vi "FindMutationByVerIndex.vi"(8 "error in (no error)":errorcluster, 9 "Old Name Index":u8, 10 "Library Version":T3, 11 "Mutation History":T4 {"LabVIEW Version" format="%.0x"}) -> (0 "error out":errorcluster, 1 "BlueSerializableVersion":T1, 2 "Mutation Record":T2 {"LabVIEW Version" format="%.0x"})   [LabVIEW 2019, in "BlueSerialization.lvlib" / "BlueSerializer.lvclass"]
uses:
  BlueSerializer.lvclass
  <vilib>/Utility/EditLVLibs/LVClass/Mutation History.ctl
  <vilib>/Utility/EditLVLibs/LVClass/Mutation Record.ctl
  <vilib>/Utility/EditLVLibs/LibVersion.ctl
  BlueSerializableVersion.ctl
  <resource>/Framework/Providers/BlueSerializationProviderShared/UserCommentToVersion.vi
  <vilib>/Utility/error.llb/Error Cluster From Error Code.vi
  <vilib>/ErrorRing/Error Ring.xnode
  <resource>/Framework/Providers/BlueSerializationProviderShared/BlueSerializationProviderShared.lvlib
  <vilib>/Utility/EditLVLibs/Edit LVLibs.lvlib
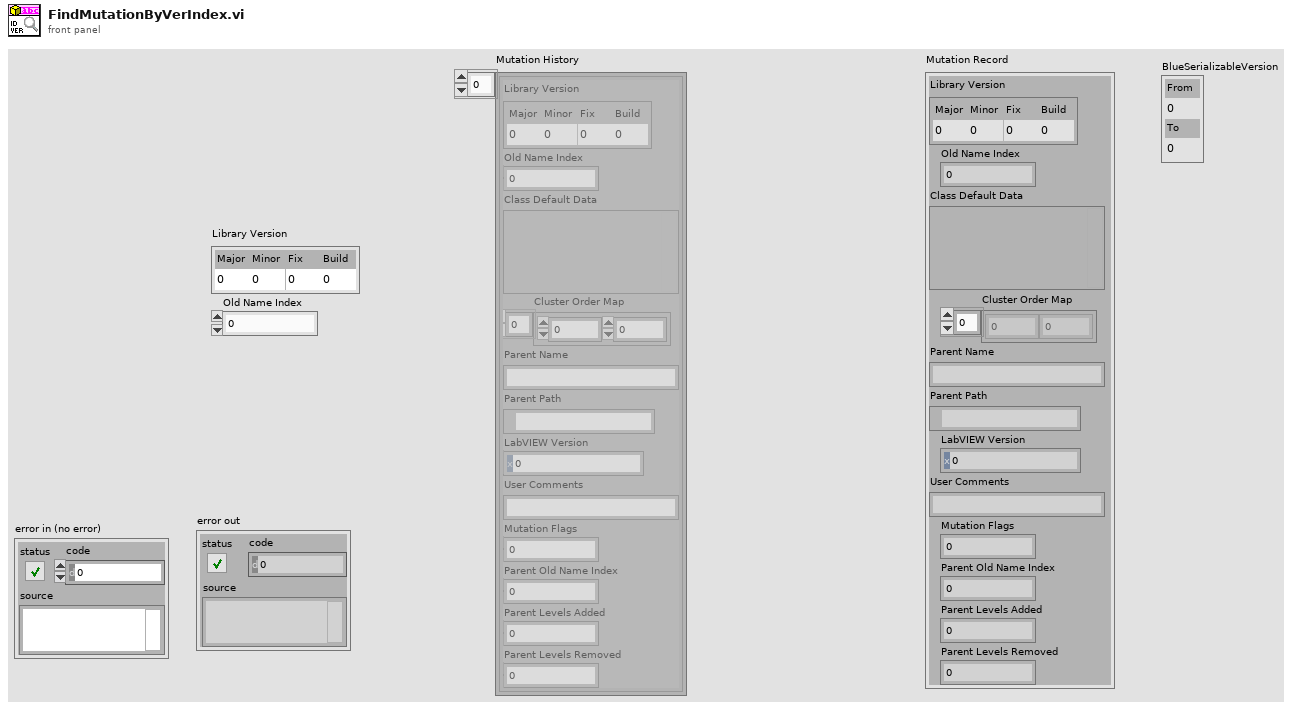
[diagram p1: front panel]
types:
  T1 = typedef "BlueSerialization.lvlib/BlueSerializer.lvclass/BlueSerializableVersion.ctl" = cluster{"From":u16, "To":u16}
  T2 = typedef "Edit LVLibs.lvlib/Mutation Record.ctl" = cluster{"Library Version":T3, "Old Name Index":u8, "Class Default Data":variant, "Cluster Order Map":u32[], "Parent Name":string, "Parent Path":path, "LabVIEW Version":u32, "User Comments":string, "Mutation Flags":u8, "Parent Old Name Index":u8, "Parent Levels Added":u16, "Parent Levels Removed":u16}
  T3 = typedef "Edit LVLibs.lvlib/LibVersion.ctl" = cluster{"Major":u16, "Minor":u16, "Fix":u16, "Build":u16}
  T4 = typedef "Edit LVLibs.lvlib/Mutation History.ctl" = T2[]
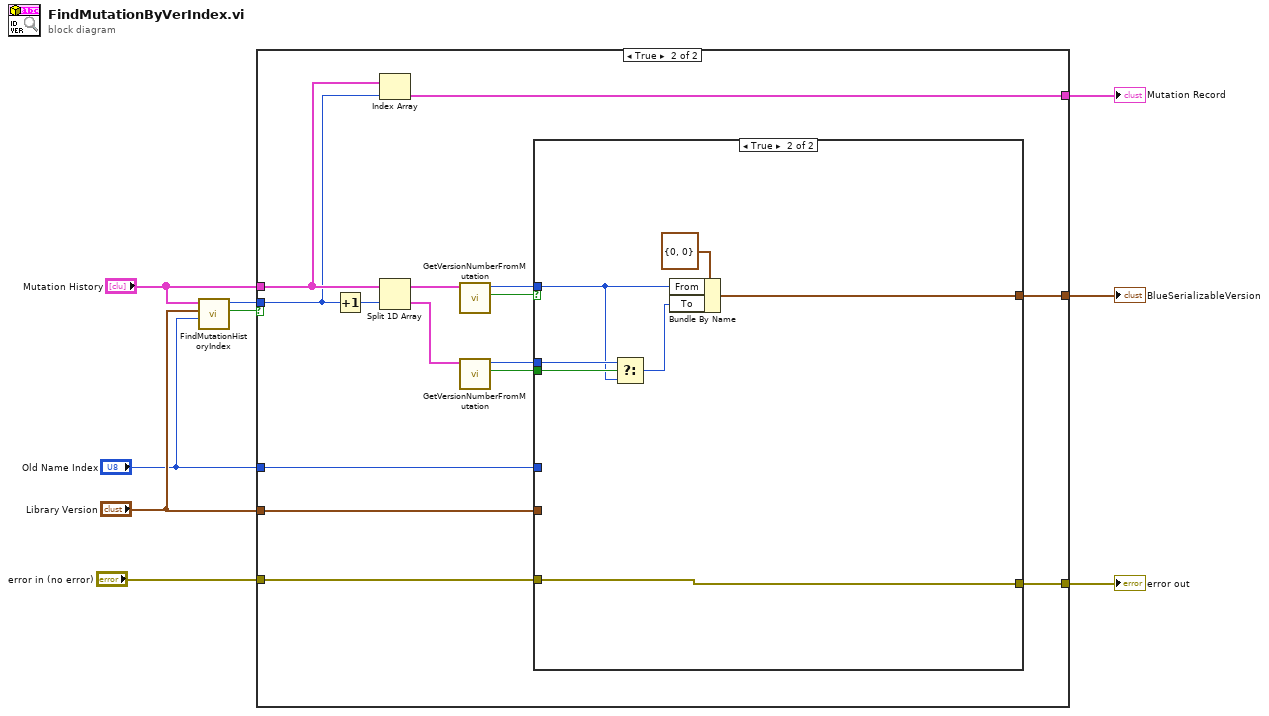
[diagram p0: block diagram]
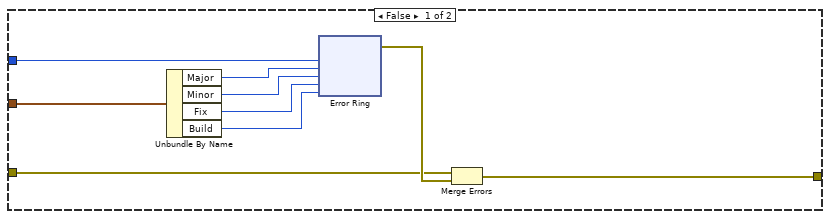
[diagram p2: hidden frame]
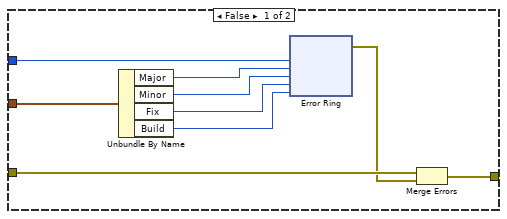
[diagram p3: hidden frame]
diagram:
  n1 = call <resource>:"FindMutationHistoryIndex.vi"("Old Name Index"="Old Name Index", "Library Version"="Library Version", "Mutation History"="Mutation History") -> ("Found?"=w3:bool, "Index"=w4:i32)  [unwired: 7 in]
  n2 = case shown="True" w3 {
    tunnel: "Library Version" -> [w18 w42]
    tunnel: "error in (no error)" -> [w12 w41]
    tunnel: [w11 w40] -> w8
    tunnel: w4 -> [_ w38]
    tunnel: "Mutation History" -> [_ w43]
    tunnel: [_ w44] -> w7
    tunnel: [_ w39] -> w6
    tunnel: "Old Name Index" -> [w10 w30]
    frame False {
      n3 = Unbundle By Name(w18) -> ("Major"=w17:u16, "Minor"=w16:u16, "Fix"=w15:u16, "Build"=w14:u16)
      n4 = xnode "Error Ring"("parameter 0"=w10, "parameter 1"=w17, "parameter 2"=w16, "parameter 3"=w15, "parameter 4"=w14) -> ("error out"=w13:errorcluster)
      n5 = Merge Errors(w12, w13) -> (w11:errorcluster)
    }
    frame True {
      n6 = Increment(x=w38) -> (x+1=w37:i32)
      n7 = Index Array(array=w43, index=w38) -> (element=w44:T2)
      n8 = Split 1D Array(array=w43, index=w37) -> (first subarray=w36:T4, second subarray=w31:T4)
      n9 = call <resource>:"GetVersionNumberFromMutation.vi"("Mutation History"=w36) -> ("BlueSerializableVersion found?"=w34:bool, "BlueSerializableVersion"=w35:u16)  [unwired: 9 in]
      n10 = call <resource>:"GetVersionNumberFromMutation.vi"("Mutation History"=w31) -> ("BlueSerializableVersion found?"=w32:bool, "BlueSerializableVersion"=w33:u16)  [unwired: 9 in]
      n11 = case shown="True" w34 {
        tunnel: w32 -> [_ w70]
        tunnel: w35 -> [_ w68]
        tunnel: w33 -> [_ w69]
        tunnel: w42 -> [w49 _]
        tunnel: w41 -> [w48 w66]
        tunnel: [w46 w66] -> w40
        tunnel: [_ w65] -> w39
        tunnel: w30 -> [w45 _]
        frame False {
          n12 = Unbundle By Name(w49) -> ("Major"=w53:u16, "Minor"=w52:u16, "Fix"=w51:u16, "Build"=w50:u16)
          n13 = xnode "Error Ring"("parameter 0"=w45, "parameter 1"=w53, "parameter 2"=w52, "parameter 3"=w51, "parameter 4"=w50) -> ("error out"=w47:errorcluster)
          n14 = Merge Errors(w48, w47) -> (w46:errorcluster)
        }
        frame True {
          n15 = Select(t=w69, s=w70, f=w68) -> (s? t:f=w67:u16)
          n16 = Bundle By Name(cluster=T1 {"From"=0, "To"=0} ("Cluster"), "From"=w68, "To"=w67) -> (w65:T1)
        }
      }
    }
  }
  "Mutation Record" <- w7
  "error out" <- w8
  "BlueSerializableVersion" <- w6
